vi "Reactor-1.vi"() -> ()   [LabVIEW 2022 SP3]
panel:
  out "T8":dbl
  in  "Condenser":bool
  in  "Income":bool
  in  "Bypass":bool
  out "Condenser_valve":bool
  out "bypass_valve":bool
  out "T7":dbl
  out "P2":dbl
  out "T6":dbl
  out "P1":dbl
  out "T1":dbl
  out "Cooling_in_valve":bool
  out "Cooling_out_valve":bool
  out "Gas_income_valve":bool
  out "T3":dbl
  out "T5":dbl
  out "T4":dbl
  out "T2":dbl
  out "Measure_H2":dbl
  in  "Setpoint_H2":dbl
  out "Measure_N2":dbl
  in  "Setpoint_N2":dbl
  out "Measure_CO2":dbl
  in  "Setpoint_CO2":dbl
  # "T1\nT1"
  # "°C"
  # "T7"
  # "°C"
  # "P1"
  # "bar"
  # "CO2"
  # "L/min"
  # "T2"
  # "°C"
  # "L/min"
  # "T3"
  # "°C"
  # "N2"
  # "L/min"
  # "T4"
  # "°C"
  # "L/min"
  # "T5"
  # "°C"
  # "H2"
  # "L/min"
  # "L/min"
  # "T8"
  # "°C"
  # "T6\nT6"
  # "°C"
  # "P2"
  # "bar"
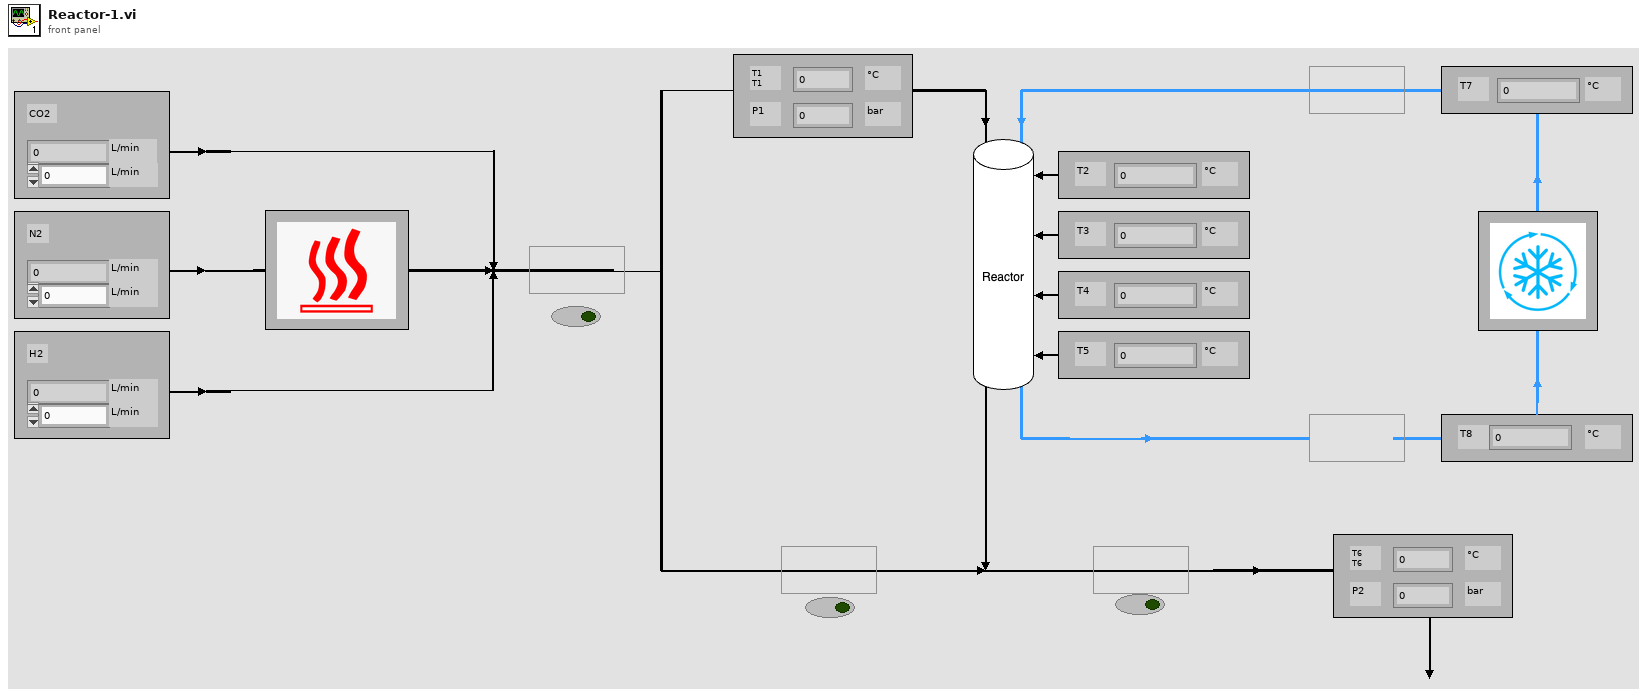
[diagram p1: front panel]
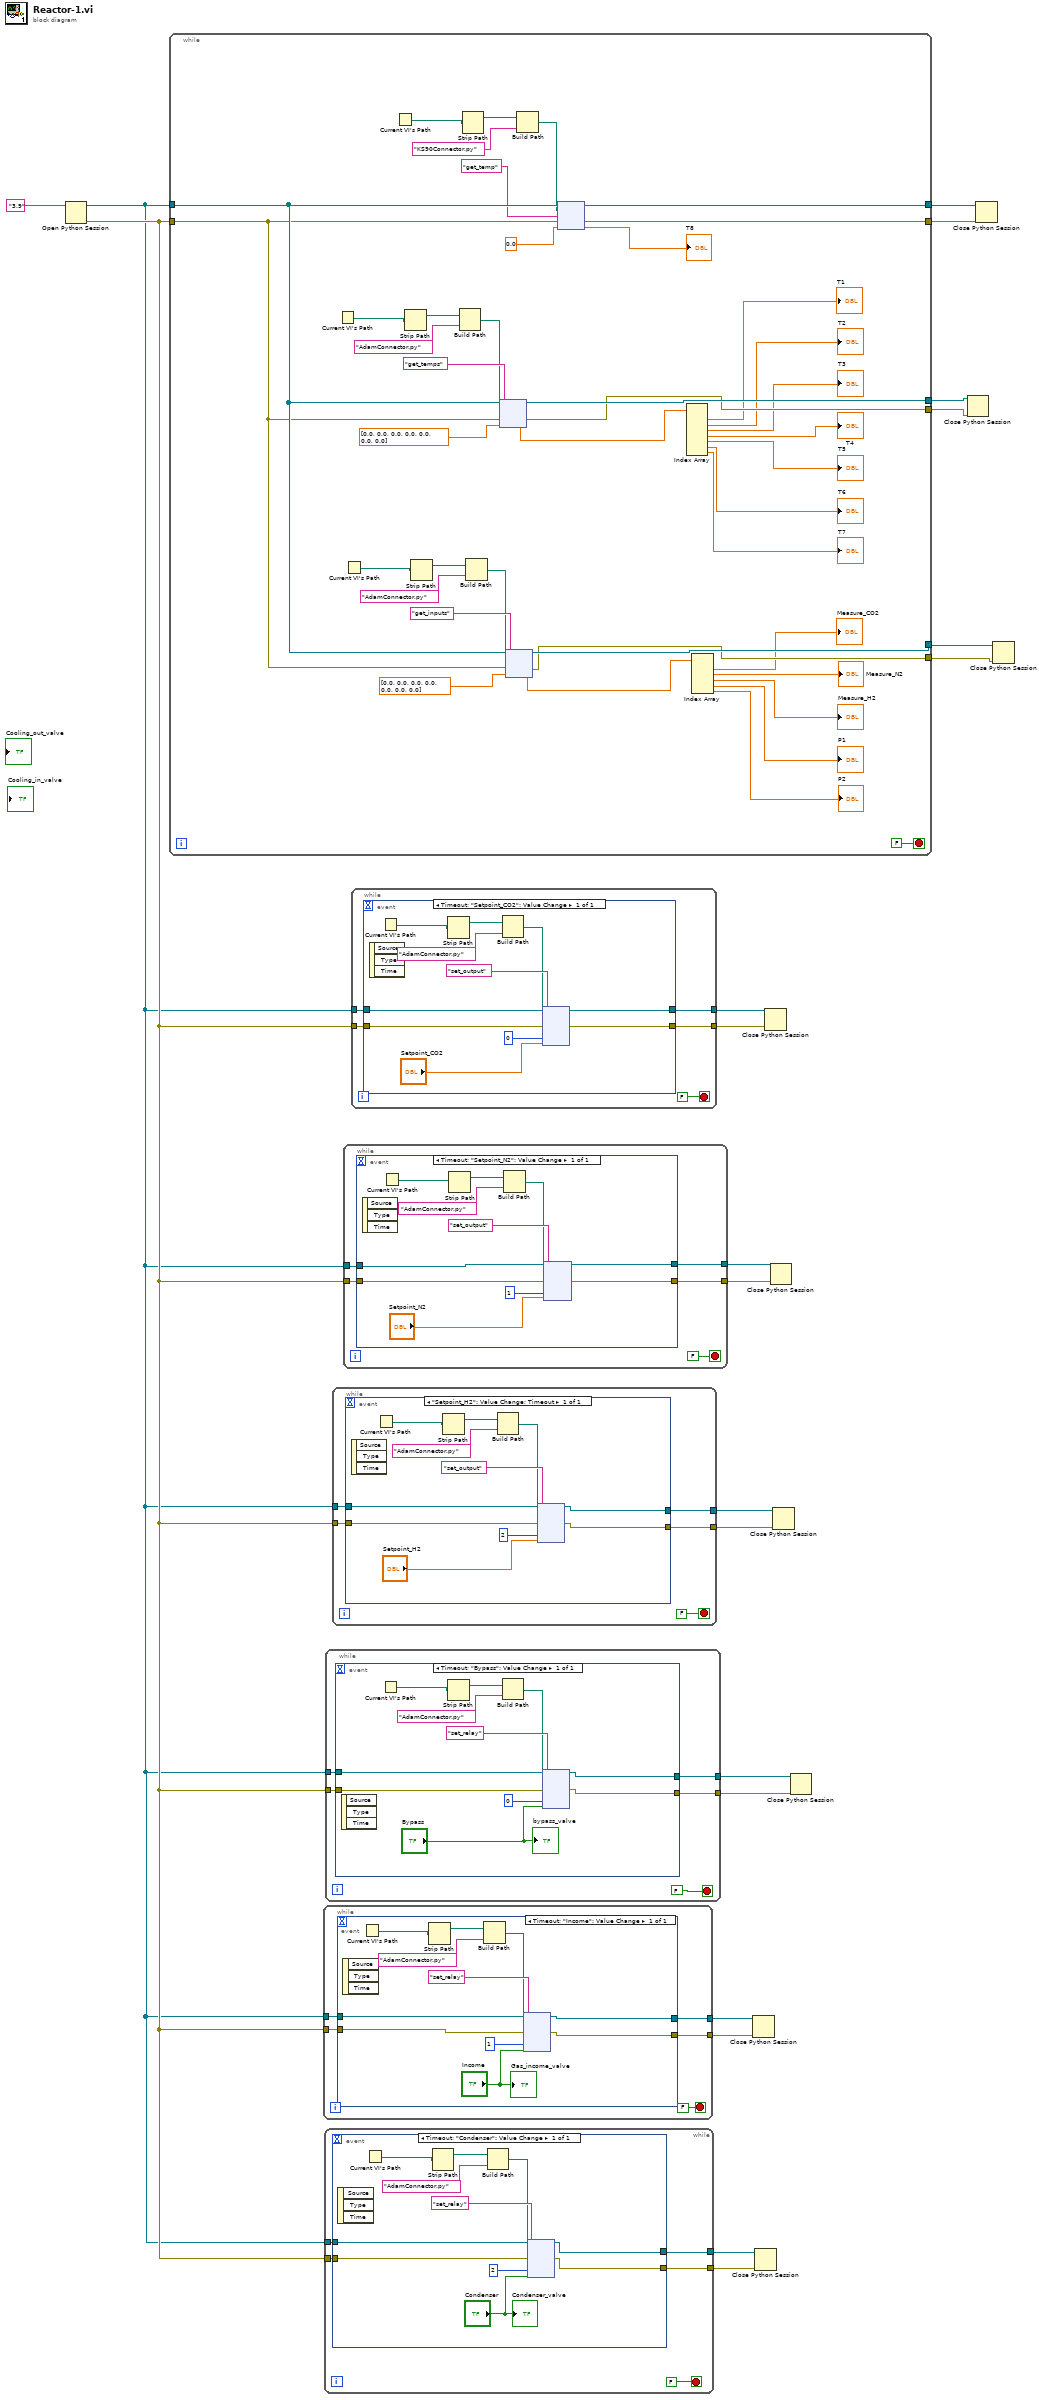
[diagram p0: block diagram]
diagram:
  n1 = Open Python Session(python version="3.9") -> (session out=w1:refnum<k35>, error out=w2:errorcluster)  [unwired: 2 in]
  n2 = while {
    tunnel: w1 -> [w62]
    tunnel: w2 -> [w61]
    tunnel: [w60] -> w20
    tunnel: [w59] -> w19
    tunnel: [w58] -> w18
    tunnel: [w57] -> w17
    tunnel: [w56] -> w16
    tunnel: [w55] -> w15
    stop <- FALSE stop-if-true
    n3 = Current VI's Path() -> (path=w53:path)
    n4 = Current VI's Path() -> (path=w39:path)
    n5 = Current VI's Path() -> (path=w25:path)
    n6 = Strip Path(path=w53) -> (stripped path=w52:path)  [unwired: 1 out]
    n7 = Strip Path(path=w39) -> (stripped path=w38:path)  [unwired: 1 out]
    n8 = Build Path(base path=w52, name or relative path="AdamConnector.py") -> (appended path=w51:path)
    n9 = Strip Path(path=w25) -> (stripped path=w26:path)  [unwired: 1 out]
    n10 = Build Path(base path=w38, name or relative path="AdamConnector.py") -> (appended path=w37:path)
    n11 = node(w62, w51, "get_temps", w61, dbl[] [0.0, 0.0, 0.0, 0.0, 0.0, 0.0, 0.0]) -> (w56:refnum<k35>, w55:errorcluster, w48:dbl[])  [unwired: 2 out]
    n12 = node(w62, w37, "get_inputs", w61, dbl[] [0.0, 0.0, 0.0, 0.0, 0.0, 0.0, 0.0]) -> (w60:refnum<k35>, w59:errorcluster, w34:dbl[])  [unwired: 2 out]
    n13 = Build Path(base path=w26, name or relative path="KS90Connector.py") -> (appended path=w27:path)
    n14 = node(w62, w27, "get_temp", w61, 0.0) -> (w58:refnum<k35>, w57:errorcluster, →"T8":dbl)  [unwired: 2 out]
    n15 = Index Array(array=w48) -> (element #1=→"T1":dbl, element #2=→"T2":dbl, element #3=→"T3":dbl, element #4=→"T4":dbl, element #5=→"T5":dbl, element #6=→"T6":dbl, element #7=→"T7":dbl)  [unwired: 7 in]
    n16 = Index Array(array=w34) -> (element #1=→"Measure_CO2":dbl, element #2=→"Measure_N2":dbl, element #3=→"Measure_H2":dbl, element #4=→"P1":dbl, element #5=→"P2":dbl)  [unwired: 5 in]
  }
  n17 = while {
    tunnel: [w67] -> w6
    tunnel: [w66] -> w5
    tunnel: w2 -> [w65]
    tunnel: w1 -> [w64]
    stop <- FALSE stop-if-true
    n18 = event shown="[0] Timeout;  \"Income\": Value Change" {
      selector: _ -> [_]
      dyn-events: _ -> [_]
      timeout: _ -> [_]
      tunnel: [w72] -> w67
      tunnel: [w71] -> w66
      tunnel: w65 -> [w70]
      tunnel: w64 -> [w69]
      event Timeout; "Income": Value Change {
        n19 = event-data() -> ()  [unwired: 1 in, 3 out]
        n20 = Current VI's Path() -> (path=w78:path)
        n21 = Strip Path(path=w78) -> (stripped path=w77:path)  [unwired: 1 out]
        n22 = Build Path(base path=w77, name or relative path="AdamConnector.py") -> (appended path=w76:path)
        n23 = node(w69, w76, "set_relay", w70, 1, "Income") -> (w72:refnum<k35>, w71:errorcluster)  [unwired: 4 in, 2 out]
        "Gas_income_valve" <- "Income"
      }
    }
  }
  n24 = while {
    tunnel: [w83] -> w4
    tunnel: [w82] -> w3
    tunnel: w2 -> [w81]
    tunnel: w1 -> [w80]
    stop <- FALSE stop-if-true
    n25 = event shown="[0] Timeout;  \"Condenser\": Value Change" {
      selector: _ -> [_]
      dyn-events: _ -> [_]
      timeout: _ -> [_]
      tunnel: [w88] -> w83
      tunnel: [w87] -> w82
      tunnel: w81 -> [w86]
      tunnel: w80 -> [w85]
      event Timeout; "Condenser": Value Change {
        n26 = event-data() -> ()  [unwired: 1 in, 3 out]
        n27 = Current VI's Path() -> (path=w94:path)
        n28 = Strip Path(path=w94) -> (stripped path=w93:path)  [unwired: 1 out]
        n29 = Build Path(base path=w93, name or relative path="AdamConnector.py") -> (appended path=w92:path)
        n30 = node(w85, w92, "set_relay", w86, 2, "Condenser") -> (w88:refnum<k35>, w87:errorcluster)  [unwired: 4 in, 2 out]
        "Condenser_valve" <- "Condenser"
      }
    }
  }
  n31 = while {
    tunnel: w2 -> [w99]
    tunnel: w1 -> [w98]
    tunnel: [w97] -> w14
    tunnel: [w96] -> w13
    stop <- FALSE stop-if-true
    n32 = event shown="[0] Timeout;  \"Bypass\": Value Change" {
      selector: _ -> [_]
      dyn-events: _ -> [_]
      timeout: _ -> [_]
      tunnel: w99 -> [w104]
      tunnel: w98 -> [w103]
      tunnel: [w102] -> w97
      tunnel: [w101] -> w96
      event Timeout; "Bypass": Value Change {
        n33 = event-data() -> ()  [unwired: 1 in, 3 out]
        n34 = Current VI's Path() -> (path=w110:path)
        n35 = Strip Path(path=w110) -> (stripped path=w109:path)  [unwired: 1 out]
        n36 = Build Path(base path=w109, name or relative path="AdamConnector.py") -> (appended path=w108:path)
        n37 = node(w103, w108, "set_relay", w104, 0, "Bypass") -> (w102:refnum<k35>, w101:errorcluster)  [unwired: 4 in, 2 out]
        "bypass_valve" <- "Bypass"
      }
    }
  }
  n38 = while {
    tunnel: [w115] -> w12
    tunnel: [w114] -> w11
    tunnel: w1 -> [w113]
    tunnel: w2 -> [w112]
    stop <- FALSE stop-if-true
    n39 = event shown="[0] \"Setpoint_H2\": Value Change;  Timeout" {
      selector: _ -> [_]
      dyn-events: _ -> [_]
      timeout: _ -> [_]
      tunnel: [w120] -> w115
      tunnel: [w119] -> w114
      tunnel: w113 -> [w118]
      tunnel: w112 -> [w117]
      event "Setpoint_H2": Value Change; Timeout {
        n40 = event-data() -> ()  [unwired: 1 in, 3 out]
        n41 = Current VI's Path() -> (path=w126:path)
        n42 = Strip Path(path=w126) -> (stripped path=w125:path)  [unwired: 1 out]
        n43 = Build Path(base path=w125, name or relative path="AdamConnector.py") -> (appended path=w124:path)
        n44 = node(w118, w124, "set_output", w117, 2, "Setpoint_H2") -> (w120:refnum<k35>, w119:errorcluster)  [unwired: 4 in, 2 out]
      }
    }
  }
  n45 = while {
    tunnel: [w131] -> w10
    tunnel: [w130] -> w9
    tunnel: w1 -> [w129]
    tunnel: w2 -> [w128]
    stop <- FALSE stop-if-true
    n46 = event shown="[0] Timeout;  \"Setpoint_N2\": Value Change" {
      selector: _ -> [_]
      dyn-events: _ -> [_]
      timeout: _ -> [_]
      tunnel: [w136] -> w131
      tunnel: [w135] -> w130
      tunnel: w129 -> [w134]
      tunnel: w128 -> [w133]
      event Timeout; "Setpoint_N2": Value Change {
        n47 = event-data() -> ()  [unwired: 1 in, 3 out]
        n48 = Current VI's Path() -> (path=w142:path)
        n49 = Strip Path(path=w142) -> (stripped path=w141:path)  [unwired: 1 out]
        n50 = Build Path(base path=w141, name or relative path="AdamConnector.py") -> (appended path=w140:path)
        n51 = node(w134, w140, "set_output", w133, 1, "Setpoint_N2") -> (w136:refnum<k35>, w135:errorcluster)  [unwired: 4 in, 2 out]
      }
    }
  }
  n52 = while {
    tunnel: [w147] -> w8
    tunnel: [w146] -> w7
    tunnel: w1 -> [w145]
    tunnel: w2 -> [w144]
    stop <- FALSE stop-if-true
    n53 = event shown="[0] Timeout;  \"Setpoint_CO2\": Value Change" {
      selector: _ -> [_]
      dyn-events: _ -> [_]
      timeout: _ -> [_]
      tunnel: [w152] -> w147
      tunnel: [w151] -> w146
      tunnel: w145 -> [w150]
      tunnel: w144 -> [w149]
      event Timeout; "Setpoint_CO2": Value Change {
        n54 = event-data() -> ()  [unwired: 1 in, 3 out]
        n55 = Current VI's Path() -> (path=w158:path)
        n56 = Strip Path(path=w158) -> (stripped path=w157:path)  [unwired: 1 out]
        n57 = Build Path(base path=w157, name or relative path="AdamConnector.py") -> (appended path=w156:path)
        n58 = node(w150, w156, "set_output", w149, 0, "Setpoint_CO2") -> (w152:refnum<k35>, w151:errorcluster)  [unwired: 4 in, 2 out]
      }
    }
  }
  n59 = Close Python Session(session in=w6, error in=w5) -> ()  [unwired: 1 out]
  n60 = Close Python Session(session in=w4, error in=w3) -> ()  [unwired: 1 out]
  n61 = Close Python Session(session in=w8, error in=w7) -> ()  [unwired: 1 out]
  n62 = Close Python Session(session in=w10, error in=w9) -> ()  [unwired: 1 out]
  n63 = Close Python Session(session in=w12, error in=w11) -> ()  [unwired: 1 out]
  n64 = Close Python Session(session in=w14, error in=w13) -> ()  [unwired: 1 out]
  n65 = Close Python Session(session in=w16, error in=w15) -> ()  [unwired: 1 out]
  n66 = Close Python Session(session in=w18, error in=w17) -> ()  [unwired: 1 out]
  n67 = Close Python Session(session in=w20, error in=w19) -> ()  [unwired: 1 out]
